vi "Start Loop.vi"(5 "C space":refnum<vi>, 7 "D space":refnum<vi>, 11 "error in (no error)":errorcluster) -> (15 "error out":errorcluster)   [LabVIEW 2020, in "DiskSpaceMonitor.xctl"]
uses:
  DiskSpaceMonitor.xctl
  MonitorLoop.vi
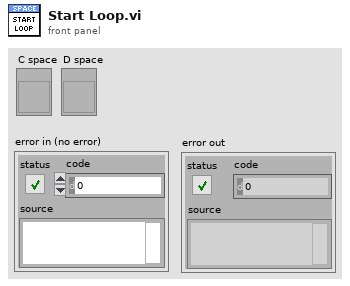
[diagram p1: front panel]
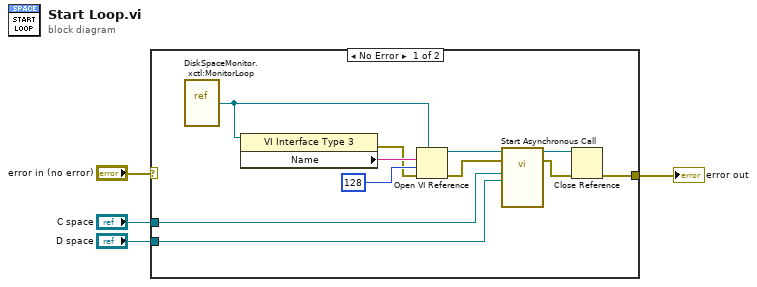
[diagram p0: block diagram]
diagram:
  n1 = case shown="No Error" "error in (no error)" {
    selector: "error in (no error)" -> [_ w16]
    tunnel: "D space" -> [w6 _]
    tunnel: "C space" -> [w7 _]
    tunnel: [w5 w16] -> w1
    frame No Error {
      n2 = vi-ref "DiskSpaceMonitor.xctl:MonitorLoop.vi"() -> (w12:refnum<vi>)
      n3 = property class="VI Interface Type 3"(reference=w12) -> (error out=w13:errorcluster, "Name"=w15:string)  [unwired: 1 in, 1 out]
      n4 = Open VI Reference(type specifier VI Refnum (for type only)=w12, vi path=w15, options=128, error in (no error)=w13) -> (vi reference=w9:refnum<vi>, error out=w8:errorcluster)  [unwired: 2 in]
      n5 = call-by-ref "Start Asynchronous Call"(reference=w9, error in=w8, "C space"=w7, "D space"=w6) -> (reference out=w11:refnum<vi>, error out=w10:errorcluster)  [unwired: 14 in]
      n6 = Close Reference(reference=w11, error in (no error)=w10) -> (error out=w5:errorcluster)
    }
    frame Error {
    }
  }
  "error out" <- w1
